vi "Initialize UniCyRO.vi"(8 "error in (no error)":errorcluster, 10 "robot ID":string, 11 "UniCyRO_Host_Sim in":refnum<class "UniCyRO_Host_Sim.lvclass">) -> (0 "error out":errorcluster, 3 "UniCyRO_Host_Sim out":refnum<class "UniCyRO_Host_Sim.lvclass">)   [LabVIEW 2012, in "UniCyRO.lvlib" / "UniCyRO_Host_Sim.lvclass"]
uses:
  UniCyRO_Host_Sim.lvclass
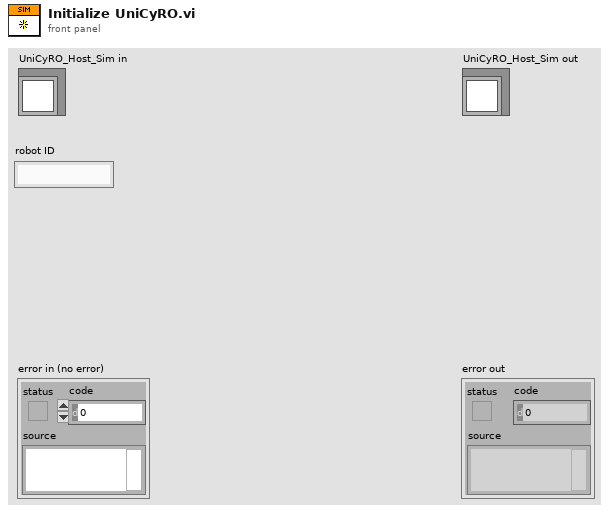
[diagram p1: front panel]
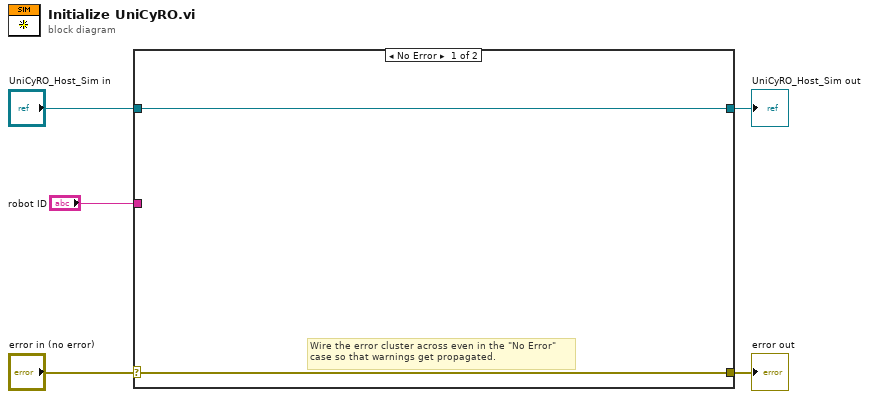
[diagram p0: block diagram]
diagram:
  n1 = case shown="No Error" "error in (no error)" {
    selector: "error in (no error)" -> [w6 w9]
    tunnel: [w6 w9] -> w4
    tunnel: [w7 w8] -> w2
    tunnel: "UniCyRO_Host_Sim in" -> [w7 w8]
    tunnel: "robot ID" -> [_ _]
    frame No Error {
      # "Wire the error cluster across even in the \"No Error\"\ncase so that warnings get propagated."
    }
    frame Error {
    }
  }
  "error out" <- w4
  "UniCyRO_Host_Sim out" <- w2
